vi "TakeOrders.vi"(8 "Error In":errorcluster, 11 "reference in":refnum<class "BubbleTeaShop.lvclass">) -> (0 "Error Out":errorcluster, 3 "reference out":refnum<class "BubbleTeaShop.lvclass">)   [LabVIEW 2020, in "BubbleTeaShop.lvclass"]
uses:
  BubbleTeaShop.lvclass
  BeverageType.ctl
  BeverageFlyweightFactory_class/BeverageFlyweightFactory.lvclass
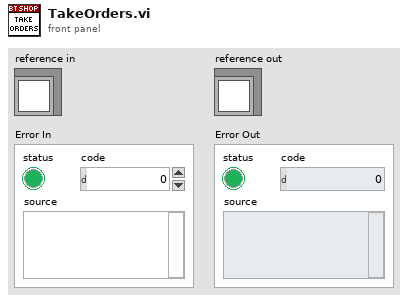
[diagram p1: front panel]
types:
  T1 = typedef "BeverageType.ctl" = enum16{"BubbleMilk", "FoamMilk", "OolongMilk", "CoconutMilk"}
  T2 = typedef "BubbleTeaShop.lvclass/ObjectAttributes.ctl" = cluster{"TakeAwayOrders":refnum<class "IBeverage.lvclass">[]}
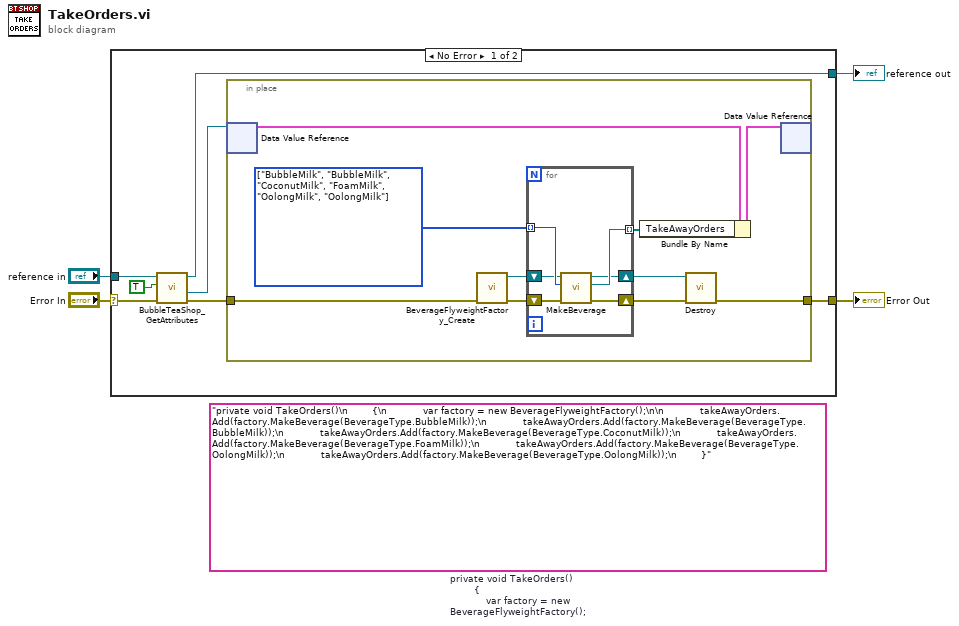
[diagram p0: block diagram]
diagram:
  (unwired) "private void TakeOrders()\n        {\n            var factory = new BeverageFlyweightFactory();\n\n            takeAwayOrders.Add(factory.MakeBeverage(BeverageType.BubbleMilk));\n            takeAwayOrders.Add(factory.MakeBeverage(BeverageType.BubbleMilk));\n            takeAwayOrders.Add(factory.MakeBeverage(BeverageType.CoconutMilk));\n            takeAwayOrders.Add(factory.MakeBeverage(BeverageType.FoamMilk));\n            takeAwayOrders.Add(factory.MakeBeverage(BeverageType.OolongMilk));\n            takeAwayOrders.Add(factory.MakeBeverage(BeverageType.OolongMilk));\n        }"  # private void TakeOrders()         {             var factory = new BeverageFlyweightFactory();              takeAwayOrders.Add(factory.MakeBeverage(BeverageType.BubbleMilk));             takeAwayOrders.Add(factory.MakeBeverage(BeverageType.BubbleMilk));             takeAwayOrders.Add(factory.MakeBeverage(BeverageType.CoconutMilk));             takeAwayOrders.Add(factory.MakeBeverage(BeverageType.FoamMilk));             takeAwayOrders.Add(factory.MakeBeverage(BeverageType.OolongMilk));             takeAwayOrders.Add(factory.MakeBeverage(BeverageType.OolongMilk));         }
  n1 = case shown="No Error" "Error In" {
    selector: "Error In" -> [w10 w29]
    tunnel: [w5 w29] -> w3
    tunnel: [w9 w28] -> w1
    tunnel: "reference in" -> [w11 w28]
    frame No Error {
      n2 = call "BubbleTeaShop_GetAttributes.vi"("error in (no error)"=w10, "OnlyGetDvrReference(False)"=TRUE, "reference in"=w11) -> ("error out"=w6:errorcluster, "DataRef"=w8:refnum<data-value>, "reference out"=w9:refnum<class "BubbleTeaShop.lvclass">)  [unwired: 5 in, 1 out]
      n3 = in-place {
        in-place-border: w6 -> [w14]
        in-place-border: [w13] -> w5
        w20 = T1[] [enum."BubbleMilk", enum."BubbleMilk", enum."CoconutMilk", enum."FoamMilk", enum."OolongMilk", enum."OolongMilk"] items=["BubbleMilk", "FoamMilk", "OolongMilk", "CoconutMilk"] ("Array")
        n4 = in-place-dvr #1(w8) -> (w12:T2)  [unwired: 1 out]
        n5 = call "BeverageFlyweightFactory_Create.vi"("Error In"=w14) -> ("Error Out"=w16:errorcluster, "reference out"=w18:refnum<class "BeverageFlyweightFactory.lvclass">)  [unwired: 9 in]
        n6 = for {
          tunnel: w20 -> [w27] mode=indexing
          tunnel: [w26] -> w19 mode=indexing
          shift-right: [w24] -> w17
          shift-left: w18 -> [w25]
          shift-right: [w22] -> w15
          shift-left: w16 -> [w23]
          n7 = call-dynamic "MakeBeverage.vi"("Error In"=w23, "Type"=w27, "reference in"=w25) -> ("Error Out"=w22:errorcluster, "Return(LabVIEW Class)"=w26:refnum<class "IBeverage.lvclass">, "reference out"=w24:refnum<class "BeverageFlyweightFactory.lvclass">)  [unwired: 6 in]
        }
        n8 = Bundle By Name(cluster=w12, "TakeAwayOrders"=w19) -> (w21:T2)
        n9 = call-dynamic "Destroy.vi"("Error In"=w15, "reference in"=w17) -> ("Error Out"=w13:errorcluster)  [unwired: 8 in, 1 out]
        n10 = in-place-dvr #1(w21) -> ()  [unwired: 2 out]
      }
    }
    frame Error {
    }
  }
  "Error Out" <- w3
  "reference out" <- w1
